vi "_BookmarkInfo to MultiCol Table.vi"(11 "BookmarkInfo":T1) -> (3 "sorted 2D array":string[][](array[string]))   [LabVIEW 2017, in "CSM_ExampleBrowser.lvlib"]
uses:
  CSM_ExampleBrowser.lvlib
  <vilib>/Utility/miscctls.llb/LVBookmarkInfoTypeDef.ctl
  f65d36f9-5bc5-4f32-83e5-176f55c1e761.vi
  <vilib>/Array/Sort 2D Array - Pop Stack.vi
  <vilib>/Array/Sort 2D Array - Push Stack.vi
  Communicable State Machine.lvlib
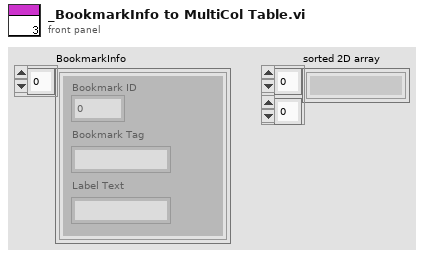
[diagram p1: front panel]
types:
  T1 = typedef "LVBookmarkInfoTypeDef.ctl" = cluster{"Bookmark ID":u32, "Bookmark Tag":string, "Label Text":string}[]
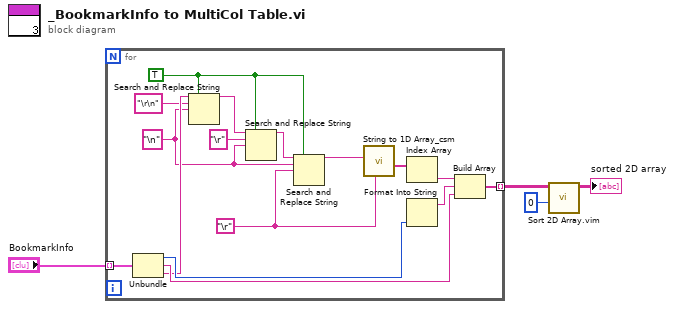
[diagram p0: block diagram]
diagram:
  n1 = for {
    tunnel: "BookmarkInfo" -> [w20] mode=indexing
    tunnel: [w17] -> w1 mode=indexing
    w9 = TRUE ("replace all? (F)")
    w11 = "\n" ("search string")
    w5 = "\r"
    n2 = Unbundle(w20) -> ("Bookmark ID"=w19:u32, "Bookmark Tag"=w16:string, "Label Text"=w15:string)
    n3 = Search and Replace String(replace all?=w9, input string=w15, search string="\r\n", replace string=w11) -> (result string=w6:string)  [unwired: 4 in, 3 out]
    n4 = Search and Replace String(replace all?=w9, input string=w6, search string="\r", replace string=w11) -> (result string=w8:string)  [unwired: 4 in, 3 out]
    n5 = Search and Replace String(replace all?=w9, input string=w8, search string=w11, replace string=w5) -> (result string=w12:string)  [unwired: 4 in, 3 out]
    n6 = call "String to 1D Array_csm.vi"("delimiter (Tab)"=w5, "string"=w12) -> ("Array of Strings"=w14:string[])  [unwired: 9 in]
    n7 = Index Array(array=w14) -> (element=w13:string)  [unwired: 1 in]
    n8 = Format Into String(w19) -> (resulting string=w18:string)  [unwired: 3 in, 1 out]
    n9 = Build Array(w13, w18, w16) -> (w17:string[])
  }
  n10 = call "Sort 2D Array.vim"("index"=0, "2D array"=w1) -> ("sorted 2D array"=→"sorted 2D array":string[][])  [unwired: 8 in, 1 out]
